vi "GetDistance.vi"(9 "Column":i32, 10 "Row":i32, 11 "MapIn":u8[][](array[numeric])) -> (2 "Score":i32)   [LabVIEW 2020, in "2022_8.lvclass"]
uses:
  2022_8.lvclass
  d6572183-c6d6-4c59-95e2-a65e9570e775.vi
  2022_8.lvclass/2022_8.ctl
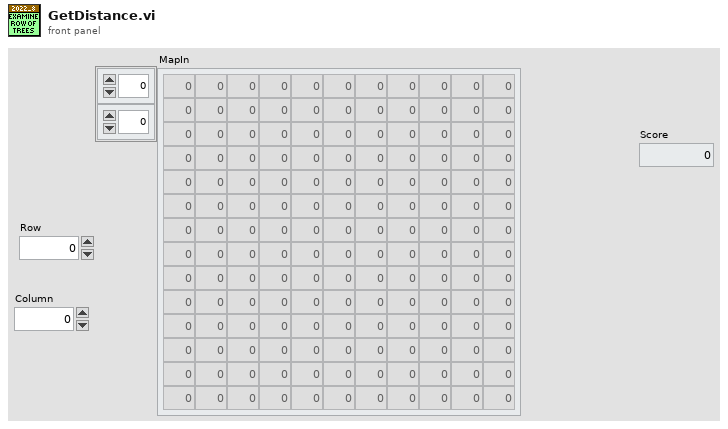
[diagram p1: front panel]
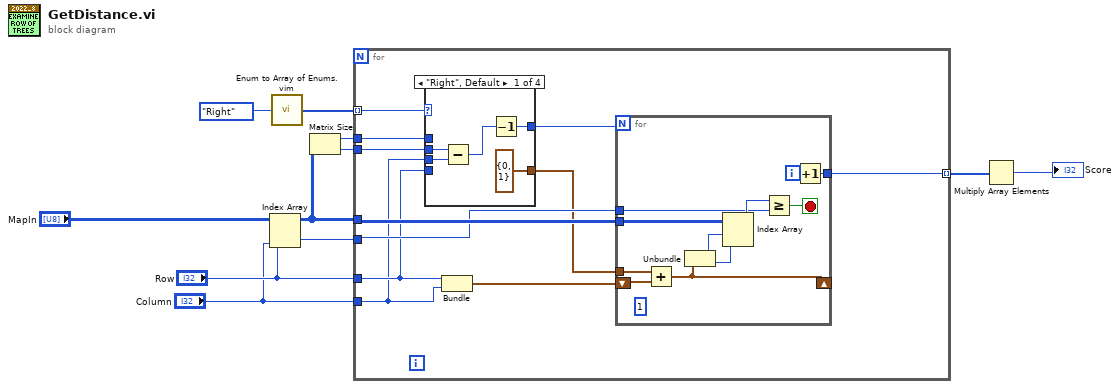
[diagram p0: block diagram]
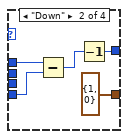
[diagram p2: hidden frame]
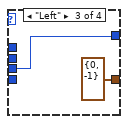
[diagram p3: hidden frame]
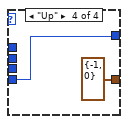
[diagram p4: hidden frame]
diagram:
  n1 = Index Array(array="MapIn", index (row)="Row", index (col)="Column") -> (element=w10:u8)
  n2 = call "Enum to Array of Enums.vim"("enum"=enum16{"Right", "Down", "Left", "Up"}."Right") -> ("array of enums"=w6:enum16{"Right", "Down", "Left", "Up"}[])
  n3 = Matrix Size(0:"MapIn") -> (1:w3:i32, 2:w4:i32)
  n4 = for {
    tunnel: w10 -> [w20]
    tunnel: "MapIn" -> [w21]
    tunnel: "Row" -> [w16]
    tunnel: "Column" -> [w15]
    tunnel: w6 -> [w19] mode=indexing
    tunnel: w4 -> [w18]
    tunnel: w3 -> [w17]
    tunnel: [w11] -> w2 mode=indexing
    n5 = case shown="\"Right\", Default" w19 {
      tunnel: w18 -> [w26 _ _ _]
      tunnel: w15 -> [w25 _ w32 _]
      tunnel: [w22 w27 w32 w34] -> w12
      tunnel: w17 -> [_ w31 _ _]
      tunnel: w16 -> [_ w30 _ w34]
      tunnel: [cluster{"Row":i32, "Column":i32} {"Row"=0, "Column"=1} ("output cluster") cluster{"Row":i32, "Column":i32} {"Row"=1, "Column"=0} ("output cluster") cluster{"Row":i32, "Column":i32} {"Row"=0, "Column"=-1} ("output cluster") cluster{"Row":i32, "Column":i32} {"Row"=-1, "Column"=0} ("output cluster")] -> w13
      frame "Right", Default {
        n6 = Subtract(x=w26, y=w25) -> (x-y=w24:i32)
        n7 = Decrement(x=w24) -> (x-1=w22:i32)
      }
      frame "Down" {
        n8 = Subtract(x=w31, y=w30) -> (x-y=w29:i32)
        n9 = Decrement(x=w29) -> (x-1=w27:i32)
      }
      frame "Left" {
      }
      frame "Up" {
      }
    }
    n10 = Bundle("Row"=w16, "Column"=w15) -> (w14:cluster{"Row":i32, "Column":i32})  [unwired: 1 in]
    n11 = for {
      N: w12 -> [_]
      tunnel: w21 -> [w46]
      tunnel: w20 -> [w44]
      shift-right: [w41] -> _
      shift-left: w14 -> [w43]
      tunnel: w13 -> [w42]
      tunnel: [w36] -> w11
      i -> [w37]
      stop <- w38 stop-if-true
      (unwired) 1 ("value")
      n12 = Add(x=w42, y=w43) -> (x+y=w41:cluster{"Row":i32, "Column":i32})
      n13 = Unbundle(w41) -> ("Row"=w40:i32, "Column"=w39:i32)
      n14 = Index Array(array=w46, index (row)=w40, index (col)=w39) -> (element=w45:u8)
      n15 = Greater Or Equal?(x=w45, y=w44) -> (x >= y?=w38:bool)
      n16 = Increment(x=w37) -> (x+1=w36:i32)
    }
  }
  n17 = Multiply Array Elements(1:w2) -> (0:→"Score":i32)
